vi "U8Arr_To_VCI_CAN_OBJ.vi"(1 "U8 Arr":u8[](array[numeric])) -> (0 "VCI_CAN_BUF_T":T1)   [LabVIEW 2011]
uses:
  _USB_CAN_SEND_BUFF_UNIT_.ctl
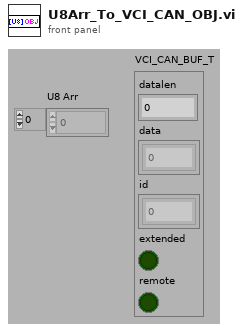
[diagram p1: front panel]
types:
  T1 = typedef "_USB_CAN_SEND_BUFF_UNIT_.ctl" = cluster{"datalen":u8, "data":u8[], "id":u8[], "extended":bool, "remote":bool}
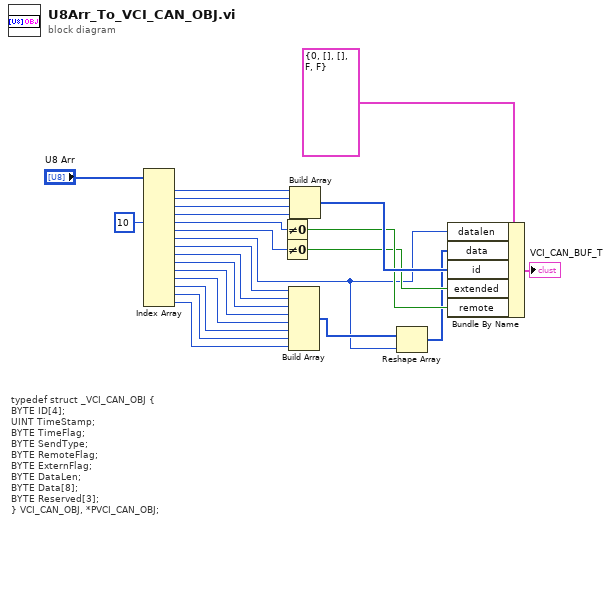
[diagram p0: block diagram]
diagram:
  # "typedef struct _VCI_CAN_OBJ { \nBYTE ID[4];\nUINT TimeStamp; \nBYTE TimeFlag;\nBYTE SendType; \nBYTE RemoteFlag; \nBYTE ExternFlag; \nBYTE DataLen; \nBYTE Data[8]; \nBYTE Reserved[3];\n} VCI_CAN_OBJ, *PVCI_CAN_OBJ;"
  n1 = Index Array(array="U8 Arr", index #5=10 ("索引")) -> (element #1=w21:u8, element #2=w20:u8, element #3=w19:u8, element #4=w18:u8, element #5=w15:u8, element #6=w13:u8, element #7=w2:u8, element #8=w11:u8, element #9=w10:u8, element #10=w9:u8, element #11=w8:u8, element #12=w7:u8, element #13=w6:u8, element #14=w5:u8, element #15=w4:u8)  [unwired: 14 in]
  n2 = Not Equal To 0?(x=w15) -> (x != 0?=w14:bool)
  n3 = Not Equal To 0?(x=w13) -> (x != 0?=w12:bool)
  n4 = Build Array(w11, w10, w9, w8, w7, w6, w5, w4) -> (w3:u8[])
  n5 = Build Array(w21, w20, w19, w18) -> (w17:u8[])
  n6 = Reshape Array(w3, w2) -> (w1:u8[])
  n7 = Bundle By Name(cluster=T1 {"datalen"=0, "data"=[], "id"=[], "extended"=FALSE, "remote"=FALSE} ("VCI_CAN_BUF_T"), "datalen"=w2, "data"=w1, "id"=w17, "extended"=w12, "remote"=w14) -> (→"VCI_CAN_BUF_T":T1)
